vi "Log Trigger.vi"(8 "error in (no error)":errorcluster, 10 "Log Trigger":bool, 11 "Embedded Data Logger System Tests in":refnum<class "Embedded Data Logger System Tests.lvclass">) -> (0 "error out":errorcluster, 3 "Embedded Data Logger System Tests out":refnum<class "Embedded Data Logger System Tests.lvclass">)   [LabVIEW 2018, in "Embedded Data Logger System Tests.lvclass"]
uses:
  Embedded Data Logger System Tests.lvclass
  C:/Dev/niveristand-custom-device-testing-tools/VeriStandTestCase/VeriStandTestCase.lvclass
  <vilib>/NI Veristand/Execution/Workspace/NI VeriStand - Set Single Channel Value.vi
  <vilib>/NI Veristand/Execution/Workspace/NI_VS Workspace ExecutionAPI.lvlib
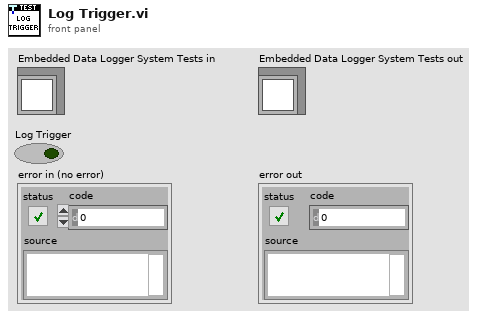
[diagram p1: front panel]
types:
  T1 = typedef "NI_VS Workspace ExecutionAPI.lvlib/WorkspaceAPI.ctl" = refnum<k24>
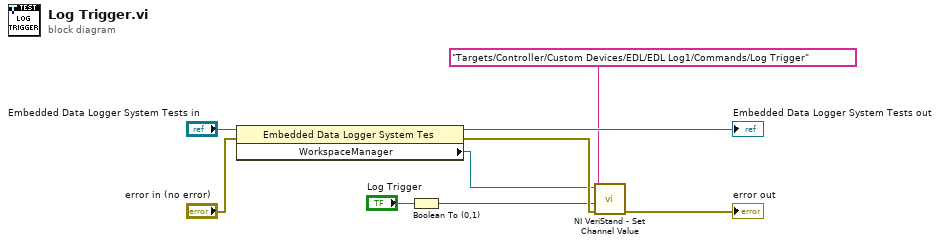
[diagram p0: block diagram]
diagram:
  n1 = property class="Embedded Data Logger System Tes"(reference="Embedded Data Logger System Tests in", error in="error in (no error)") -> (reference out=→"Embedded Data Logger System Tests out":refnum<class "Embedded Data Logger System Tests.lvclass">, error out=w6:errorcluster, "WorkspaceManager"=w5:T1)
  n2 = Boolean To (0,1)(Boolean="Log Trigger") -> (0, 1=w2:i16)
  n3 = call-poly <vilib>:"NI VeriStand - Set Channel Value.vi"("error in (no error)"=w6, "Value"=w2, "Channel"="Targets/Controller/Custom Devices/EDL/EDL Log1/Commands/Log Trigger", "WorkspaceManager in"=w5) -> ("error out"=→"error out":errorcluster)  [unwired: 6 in, 1 out]
